vi "FPGAController_v4_check_velocity.vi"() -> ()   [LabVIEW 2015]
uses:
  <vilib>/Utility/miscctls.llb/LVPointTypeDef.ctl
  <vilib>/rvi/interface/nirviOpenFPGA/nirviOpenFPGA.xnode
  <vilib>/rvi/interface/nirviMethod/nirviMethod.xnode
  <vilib>/FPGA/interface/niFpgaViExecutionMode.ctl
  <vilib>/addons/database/NI_Database_API.lvlib
  <vilib>/addons/database/Recordset.llb/Rec Fetch Recordset Data (R).vi
  <vilib>/addons/database/Connection.llb/Conn Execute.vi
  <vilib>/addons/database/Recordset.llb/Rec Destroy - Connection.vi
  <vilib>/addons/database/_DB Variant To Data/Database Variant To Data.xnode
  <vilib>/rvi/interface/nirviReadWriteControl/nirviReadWriteControl.xnode
  NiFpgaLv.dll
  <vilib>/Utility/error.llb/Error Cluster From Error Code.vi
  <vilib>/rvi/errors/niLvFpgaAdjustHostInterfaceError.vi
  <userlib>/_OpenG.lib/file/file.llb/Strip Path Extension - Path__ogtk.vi
  <vilib>/rvi/interface/nirviCloseFPGA/nirviCloseFPGA.xnode
  <vilib>/Utility/file.llb/Write Delimited Spreadsheet (DBL).vi
  <userlib>/_OpenG.lib/comparison/comparison.llb/Boolean Changed__ogtk.vi
  <userlib>/_OpenG.lib/comparison/comparison.llb/DBL Changed__ogtk.vi
  <vilib>/Utility/file.llb/Write Delimited Spreadsheet (string).vi
  FPGA Bitfiles/FPGAnew_FPGATarget_FPGAcodecheckvel_3bbhIfqrdmo.lvbitx
  <vilib>/FPGAPlugInAG/PXIe-7971R/niLvFpga_Close_PXIe-7971R.vi
  <vilib>/FPGAPlugInAG/PXIe-7971R/niLvFpga_Open_PXIe-7971R.vi
panel:
  in  "Tab Control":enum32{"Debugging", "Check Values"}(tab)
  out "Low Mass Limit":fxp<+,31,17>
  out "High Mass Limit":fxp<+,31,17>
  out "Low Charge Limit":i16
  out "High Charge Limit":i16
  out "High velocity count":i32=210
  out "Low velocity count":i32=21000
  out "time":timestamp[](array[timestamp])
  out "Velocity":dbl[](array[numeric])
  out "Filter":i16[](array[numeric])
  out "Time Betwee Shots":dbl
  in  "Min. Time\nBetween Shots (s)":dbl
  in  "Rate Limiting":bool
  out "Update Threshold":bool
  in  "Auto Threshold":bool
  in  "stop":bool
  out "stopping":bool
  in  "One Shot Mode":bool
  out "High Velocity":dbl=100000.0
  out "Low Velocity":dbl=1000.0
  out "Filter 1 Peak":i32=295996
  out "Filter 2 Peak":i32=120664
  out "Filter 3 Peak":i32=46254
  out "Filter 4 Peak":i32=18191
  out "Filter 5 Peak":i32=13910
  out "Filter 6 Peak":i32=9863
  out "Filter 7 Peak":i32=7483
  in  "Zero Peak Values":bool
  in  "Peak-Threshold Factor":dbl=2.0
  in  "Assign Threshold":bool
  in  "Filter1 Threshold":i32=-887988
  in  "Filter2 Threshold":i32=-361992
  in  "Filter3 Threshold":i32=-138762
  in  "Filter4 Threshold":i32=-54306
  in  "Filter5 Threshold":i32=-41730
  in  "Filter6 Threshold":i32=-29358
  in  "Filter7 Threshold":i32=-21165
  out "High Charge Limit (fC)":dbl=100.0
  out "Low Charge Limit (fC)":dbl
  out "Low Mass (kg)":dbl
  out "High Mass (kg)":dbl=inf
  out "Peletron (MV)":dbl=2.0
  in  "Run Mode":bool
  out "error out":errorcluster
  out "Sensitivity":dbl
  out "Last Update:":timestamp
  out "Updating FPGA":bool
  in  "Delay Ring":dbl(ring)=3.15039 items=["Ablation Chamber"=6.45, "LEIL Chamber"=4.318, "Third Detector"=3.15039, "Custom"=0.0]
  in  "Delay Value":dbl=3.0 min=0.0
  in  "Delay Name":string
  in  "Rearm Trigger":bool
  out "Armed":bool
  in  "Add Delay":bool
  in  "Raise Threshold":bool
  in  "Lower Threshold":bool
  out "Del Armed":bool
  # "Settings"
  # "Thresholds"
  # "Peaks"
  # "Independent Variable"
  # "Threshold 1"
  # "Peak 1"
  # "Low Vel."
  # "High Vel."
  # "Threshold 2"
  # "Peak 2"
  # "Low Q (fC)"
  # "High Q (fC)"
  # "Threshold 3"
  # "Peak 3"
  # "Low Mass (kg)"
  # "High Q (fC)"
  # "Threshold 4"
  # "Peak 4"
  # "Sens. (V/pC)"
  # "Peletron (MV)"
  # "Threshold 5"
  # "Peak 5"
  # "Peak Threshold Factor"
  # "Threshold 6"
  # "Peak 6"
  # "Delay Trigger"
  # "Dist. from 2nd Det. (m)"
  # "Name"
  # "Threshold 7"
  # "Peak 7"
  # "Dubugging"
  # "Plate Control While Loop Counter"
  # "Current Value of Running Average"
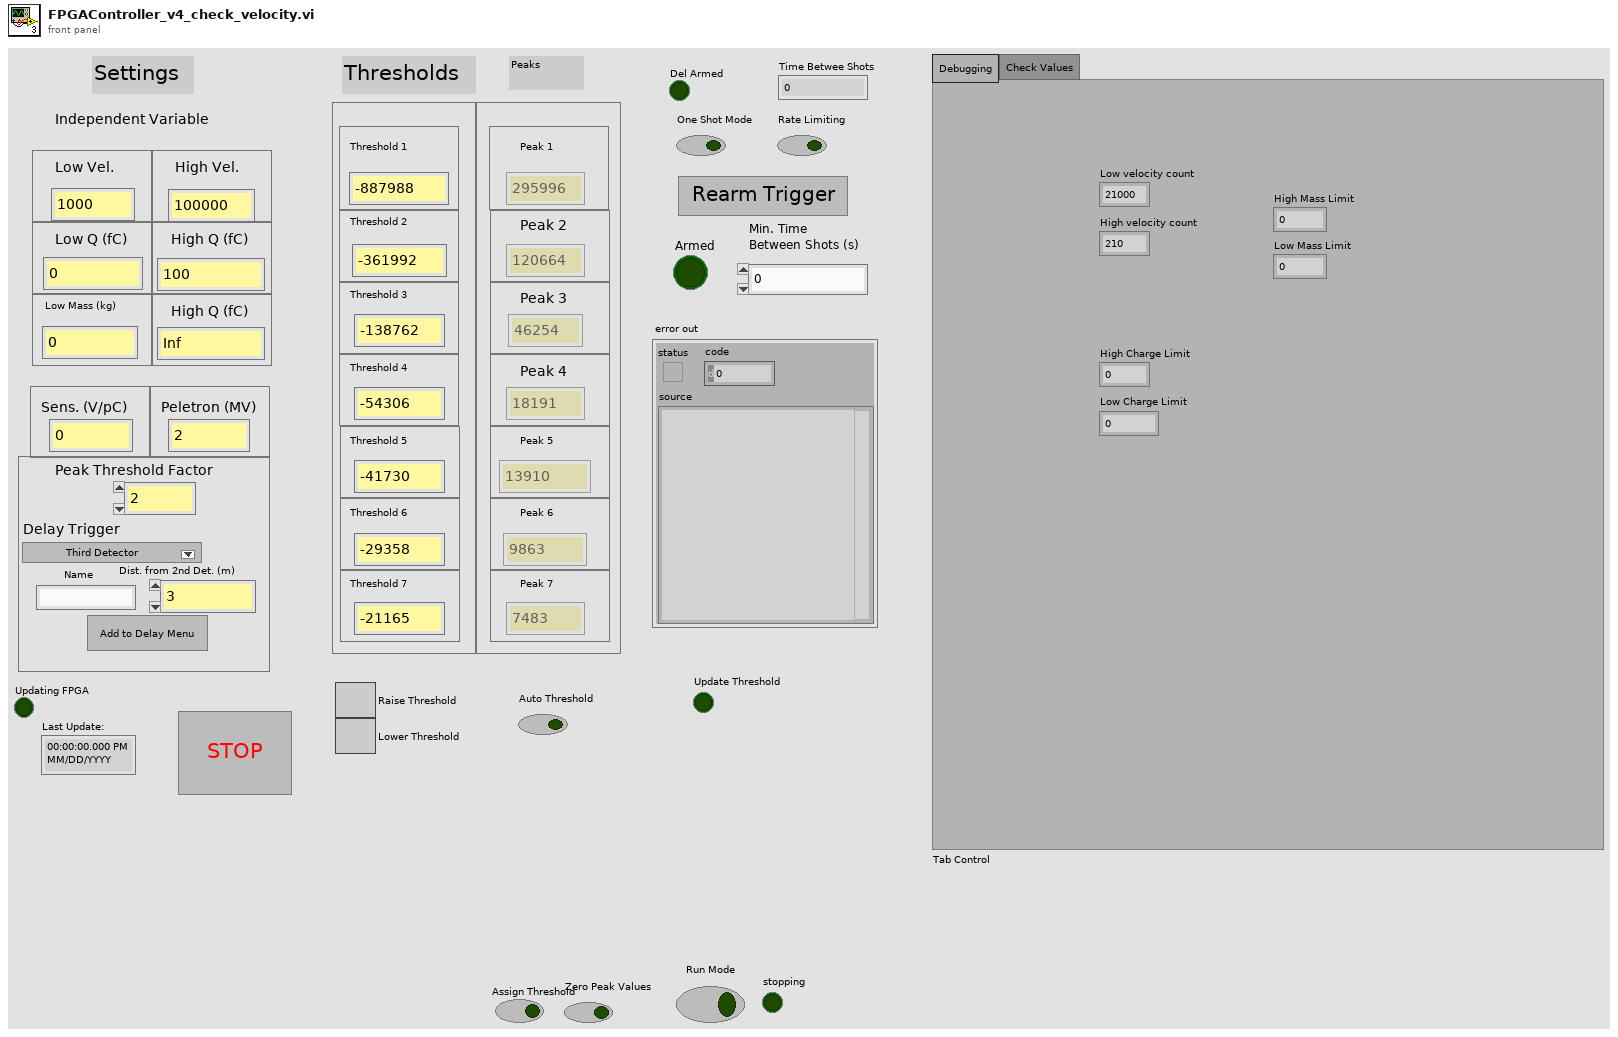
[diagram p1: front panel]
types:
  T1 = typedef "LVPointTypeDef.ctl" = cluster{"Horizontal":i16, "Vertical":i16}
  T2 = enum8{"Enabled", "Disabled", "Disabled and Grayed Out"}
  T3 = typedef "NI_Database_API.lvlib/Conn ObjectReference.ctl" = refnum<k1>
  T4 = cluster{"Filter 1 Peak":i32, "Filter 2 Peak":i32, "Filter 3 Peak":i32, "Filter 4 Peak":i32, "Filter 5 Peak":i32, "Filter 6 Peak":i32, "Filter 7 Peak":i32}
  T5 = typedef "NI_Database_API.lvlib/Rec ObjectReference.ctl" = refnum<k1>
  T6 = typedef "LVStringsAndValuesArrayTypeDef_DBL.ctl" = cluster{"String":string, "Value":dbl}[]
  T7 = cluster{"Numeric":dbl, "Numeric":dbl, "Numeric":dbl, "Numeric":dbl, "Numeric":dbl, "Numeric":dbl, dbl, dbl, "Value":dbl, fxp<+,16,7>, bool}
  T8 = cluster{"Filter 1 Detector 3 Correlation":i32, "Filter 2 Detector 3 Correlation":i32, "Filter 3 Detector 3 Correlation":i32, "Filter 4 Detector 3 Correlation":i32, "Filter 5 Detector 3 Correlation":i32, "Filter 6 Detector 3 Correlation":i32, "Filter 7 Detector 3 Correlation":i32}
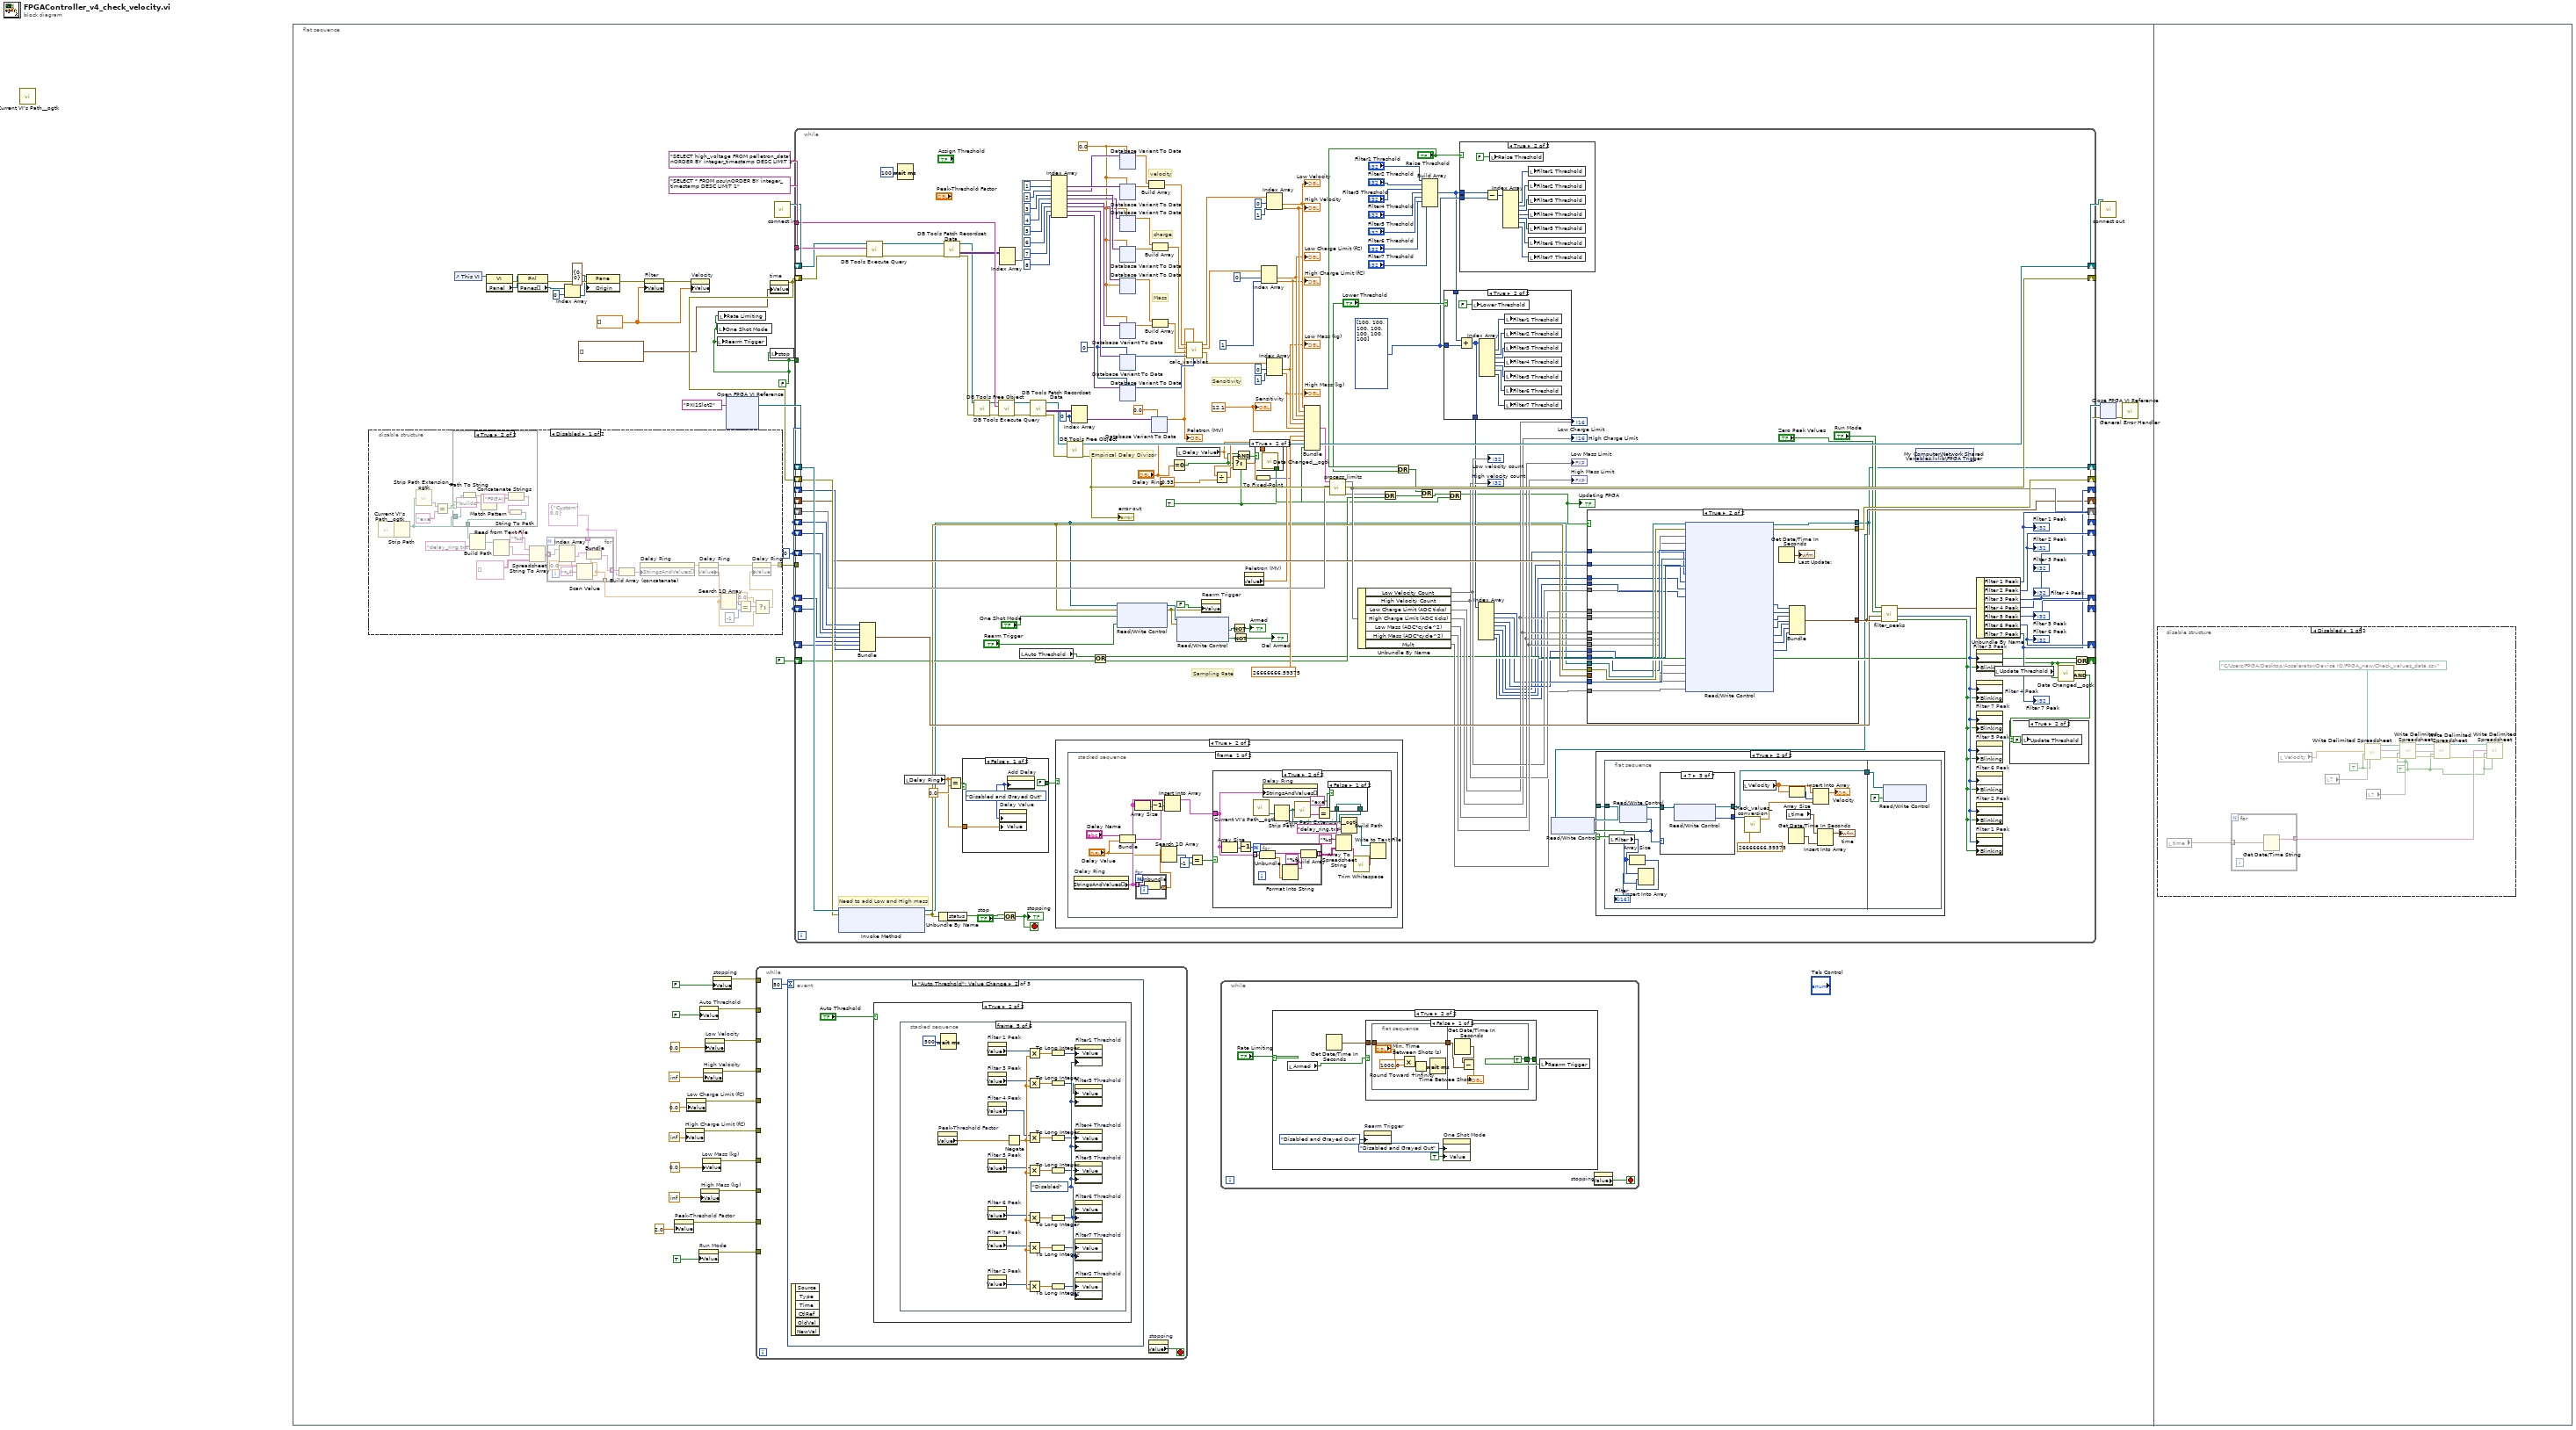
[diagram p0: block diagram]
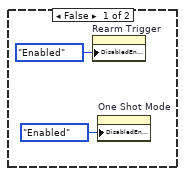
[diagram p4: hidden frame]
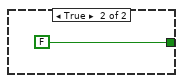
[diagram p5: hidden frame]
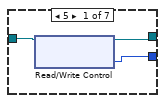
[diagram p7: hidden frame]
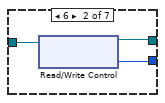
[diagram p8: hidden frame]
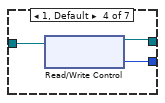
[diagram p9: hidden frame]
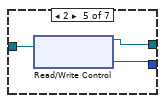
[diagram p10: hidden frame]
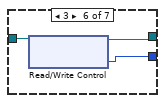
[diagram p11: hidden frame]
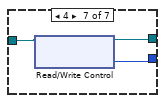
[diagram p12: hidden frame]
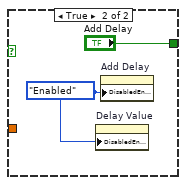
[diagram p17: hidden frame]
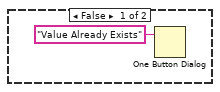
[diagram p19: hidden frame]
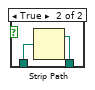
[diagram p20: hidden frame]
diagram:
  n1 = call <userlib>:"Current VI's Path__ogtk.vi"() -> ()  [unwired: 1 in, 1 out]
  n2 = flat-sequence {
    frame #0 {
      w1 = dbl[] [] ("Delay")
      w10 = FALSE
      w45 = 0
      n3 = disable-structure shown="Disabled" {
        disable-tunnel: [w53 _] -> w12
        frame Disabled {
          w62 = cluster{"String":string, "Value":dbl} {"String"="Custom", "Value"=0.0}
          n4 = call <userlib>:"Current VI's Path__ogtk.vi"() -> ("Current VI's Path (+ Relative)"=w71:path)  [unwired: 1 in]
          n5 = Strip Path(path=w71) -> (stripped path=w57:path)  [unwired: 1 out]
          n6 = call-poly <userlib>:"Strip Path Extension__ogtk.vi"("path"=w57) -> ("extension"=w61:string)  [unwired: 1 out]
          n7 = Equal?(x=w61, y="exe") -> (x = y?=w58:bool)
          n8 = case shown="True" w58 {
            tunnel: w57 -> [w80 w87]
            tunnel: [w80 w81] -> w56
            frame False {
            }
            frame True {
              n9 = Path To String(path=w87) -> (string=w86:string)
              n10 = Match Pattern(string=w86, regular expression="builds") -> (before substring=w84:string)  [unwired: 1 in, 3 out]
              n11 = Concatenate Strings(w84, "FPGA\\" ("string")) -> (w82:string)
              n12 = String To Path(string=w82) -> (path=w81:path)
            }
          }
          n13 = Build Path(base path=w56, name or relative path="delay_ring.txt") -> (appended path=w59:path)
          n14 = Read from Text File(file (use dialog)=w59) -> (text=w69:string)  [unwired: 3 in, 3 out]
          n15 = Spreadsheet String To Array(format string="%s", spreadsheet string=w69, array type (2D Dbl)=string[][] []) -> (array=w66:string[][])  [unwired: 1 in]
          n16 = for {
            tunnel: w66 -> [w79] mode=indexing
            tunnel: w62 -> [w77]
            tunnel: [w73] -> w63 mode=indexing
            tunnel: [w72] -> w55 mode=indexing
            n17 = Index Array(array=w79) -> (element #1=w78:string, element #2=w76:string)  [unwired: 2 in]
            n18 = Scan Value(string=w76, format string="%f", default (0 dbl)=0.0) -> (value=w72:dbl)  [unwired: 1 out]
            n19 = Bundle(cluster=w77, "String"=w78, "Value"=w72) -> (w73:cluster{"String":string, "Value":dbl})
          }
          n20 = Build Array (concatenate)(w63, w62) -> (w65:cluster{"String":string, "Value":dbl}[])
          n21 = property on="Delay Ring" class="Ring (strict)"("StringsAndValues[]"=w65) -> (error out=w64:errorcluster)  [unwired: 2 in, 1 out]
          n22 = property on="Delay Ring" class="Ring (strict)"(error in=w64) -> (error out=w54:errorcluster, "Value"=w48:dbl)  [unwired: 1 in, 1 out]
          n23 = Search 1D Array(1D array=w55, element=w48) -> (index of element=w52:i32)  [unwired: 1 in]
          n24 = Equal?(x=w52, y=-1) -> (x = y?=w50:bool)
          n25 = Select(t=0.0, s=w50, f=w48) -> (s? t:f=w49:dbl)
          n26 = property on="Delay Ring" class="Ring (strict)"(error in=w54, "Value"=w49) -> (error out=w53:errorcluster)  [unwired: 1 in, 1 out]
        }
        frame Enabled {
        }
      }
      n27 = control-ref of="This VI"() -> (w22:refnum<vi>)
      n28 = property class="VI"(reference=w22) -> (error out=w21:errorcluster, "Panel"=w20:refnum<vi>)  [unwired: 1 in, 1 out]
      n29 = property class="Pnl"(reference=w20, error in=w21) -> (error out=w19:errorcluster, "Panes[]"=w18:refnum<vi>[])  [unwired: 1 out]
      n30 = Index Array(array=w18, index=0) -> (element=w16:refnum<vi>)
      n31 = property class="Pane"(reference=w16, error in=w19, "Origin"=T1 {"Horizontal"=0, "Vertical"=0}) -> (error out=w3:errorcluster)  [unwired: 1 out]
      n32 = property on="Filter" class="Arr (strict)"(error in=w3, "Value"=w1) -> (error out=w2:errorcluster)  [unwired: 1 in, 1 out]
      n33 = property on="Peak-Threshold Factor" class="DigNum (strict)"("Value"=2.0 ("Peak-Threshold Factor")) -> (error out=w6:errorcluster)  [unwired: 2 in, 1 out]
      n34 = property on="High Charge Limit (fC)" class="DigNum (strict)"("Value"=inf ("High Charge Limit (fC)")) -> (error out=w32:errorcluster)  [unwired: 2 in, 1 out]
      n35 = property on="Low Charge Limit (fC)" class="DigNum (strict)"("Value"=0.0 ("Low Charge Limit (fC)")) -> (error out=w34:errorcluster)  [unwired: 2 in, 1 out]
      n36 = property on="Velocity" class="Arr (strict)"(error in=w2, "Value"=w1) -> ()  [unwired: 1 in, 2 out]
      n37 = property on="Run Mode" class="Bool (strict)"("Value"=TRUE ("Run Mode")) -> (error out=w4:errorcluster)  [unwired: 2 in, 1 out]
      n38 = property on="Auto Threshold" class="Bool (strict)"("Value"=FALSE ("Auto Threshold")) -> (error out=w40:errorcluster)  [unwired: 2 in, 1 out]
      n39 = property on="High Mass (kg)" class="DigNum (strict)"("Value"=inf ("High Mass (kg)")) -> (error out=w28:errorcluster)  [unwired: 2 in, 1 out]
      n40 = property on="Low Mass (kg)" class="DigNum (strict)"("Value"=0.0 ("Low Mass (kg)")) -> (error out=w30:errorcluster)  [unwired: 2 in, 1 out]
      n41 = property on="High Velocity" class="DigNum (strict)"("Value"=inf ("High Velocity")) -> (error out=w36:errorcluster)  [unwired: 2 in, 1 out]
      n42 = property on="Low Velocity" class="DigNum (strict)"("Value"=0.0 ("Low Velocity")) -> (error out=w38:errorcluster)  [unwired: 2 in, 1 out]
      n43 = property on="stopping" class="Bool (strict)"("Value"=FALSE ("stopping")) -> (error out=w42:errorcluster)  [unwired: 2 in, 1 out]
      n44 = local write "Rearm Trigger"(w10) -> ()
      n45 = local write "One Shot Mode"(w10) -> ()
      n46 = local write "Rate Limiting"(w10) -> ()
      n47 = xnode "Open FPGA VI Reference"("resource name"=tag "PXI1Slot2") -> ("FPGA VI Reference Out"=w14:refnum<k20>)  [unwired: 1 in, 1 out]
      n48 = while {
        tunnel: w42 -> [_]
        tunnel: w40 -> [_]
        tunnel: w38 -> [_]
        tunnel: w36 -> [_]
        tunnel: w34 -> [_]
        tunnel: w32 -> [_]
        tunnel: w30 -> [_]
        tunnel: w28 -> [_]
        tunnel: w6 -> [_]
        tunnel: w4 -> [_]
        stop <- w710 stop-if-true
        n49 = event shown="[1] \"Auto Threshold\": Value Change" {
          selector: _ -> [_ _ _]
          dyn-events: _ -> [_ _ _]
          timeout: 50 -> [_ _ _]
          event Timeout {
            n50 = event-data() -> ()  [unwired: 1 in, 2 out]
          }
          event "Auto Threshold": Value Change {
            n51 = event-data() -> ()  [unwired: 1 in, 6 out]
            n52 = case shown="True" "Auto Threshold" {
              frame False {
                w712 = T2."Enabled" ("Disabled")
                n53 = property on="Filter1 Threshold" class="DigNum (strict)"("DisabledEnum"=w712) -> ()  [unwired: 2 in, 2 out]
                n54 = property on="Filter2 Threshold" class="DigNum (strict)"("DisabledEnum"=w712) -> ()  [unwired: 2 in, 2 out]
                n55 = property on="Filter3 Threshold" class="DigNum (strict)"("DisabledEnum"=w712) -> ()  [unwired: 2 in, 2 out]
                n56 = property on="Filter4 Threshold" class="DigNum (strict)"("DisabledEnum"=w712) -> ()  [unwired: 2 in, 2 out]
                n57 = property on="Filter5 Threshold" class="DigNum (strict)"("DisabledEnum"=w712) -> ()  [unwired: 2 in, 2 out]
                n58 = property on="Filter6 Threshold" class="DigNum (strict)"("DisabledEnum"=w712) -> ()  [unwired: 2 in, 2 out]
                n59 = property on="Filter7 Threshold" class="DigNum (strict)"("DisabledEnum"=w712) -> ()  [unwired: 2 in, 2 out]
              }
              frame True {
                n60 = stacked-sequence {
                  frame #0 {
                    n61 = property on="Zero Peak Values" class="Bool (strict)"("Value"=TRUE ("Zero Peak Values")) -> ()  [unwired: 2 in, 2 out]
                    n62 = property on="Run Mode" class="Bool (strict)"("Value"=FALSE ("Run Mode")) -> ()  [unwired: 2 in, 2 out]
                  }
                  frame #1 {
                    n63 = Wait (ms)(milliseconds to wait=u32 2000) -> ()  [unwired: 1 out]
                  }
                  frame #2 {
                    n64 = property on="Zero Peak Values" class="Bool (strict)"("Value"=FALSE ("Zero Peak Values")) -> ()  [unwired: 2 in, 2 out]
                  }
                  frame #3 {
                    n65 = Wait (ms)(milliseconds to wait=u32 8000) -> ()  [unwired: 1 out]
                  }
                  frame #4 {
                    w742 = T2."Disabled" ("Disabled")
                    n66 = property on="Peak-Threshold Factor" class="DigNum (strict)"() -> ("Value"=w727:dbl)  [unwired: 2 in, 2 out]
                    n67 = Wait (ms)(milliseconds to wait=u32 500) -> ()  [unwired: 1 out]
                    n68 = property on="Filter 1 Peak" class="DigNum (strict)"() -> ("Value"=w725:i32)  [unwired: 2 in, 2 out]
                    n69 = property on="Filter 3 Peak" class="DigNum (strict)"() -> ("Value"=w723:i32)  [unwired: 2 in, 2 out]
                    n70 = property on="Filter 4 Peak" class="DigNum (strict)"() -> ("Value"=w722:i32)  [unwired: 2 in, 2 out]
                    n71 = property on="Filter 5 Peak" class="DigNum (strict)"() -> ("Value"=w721:i32)  [unwired: 2 in, 2 out]
                    n72 = property on="Filter 6 Peak" class="DigNum (strict)"() -> ("Value"=w720:i32)  [unwired: 2 in, 2 out]
                    n73 = property on="Filter 7 Peak" class="DigNum (strict)"() -> ("Value"=w719:i32)  [unwired: 2 in, 2 out]
                    n74 = property on="Filter 2 Peak" class="DigNum (strict)"() -> ("Value"=w724:i32)  [unwired: 2 in, 2 out]
                    n75 = Negate(x=w727) -> (-x=w726:dbl)
                    n76 = Multiply(x=w725, y=w726) -> (x*y=w741:dbl)
                    n77 = Multiply(x=w723, y=w726) -> (x*y=w737:dbl)
                    n78 = Multiply(x=w722, y=w726) -> (x*y=w735:dbl)
                    n79 = Multiply(x=w721, y=w726) -> (x*y=w733:dbl)
                    n80 = Multiply(x=w720, y=w726) -> (x*y=w731:dbl)
                    n81 = Multiply(x=w719, y=w726) -> (x*y=w729:dbl)
                    n82 = Multiply(x=w724, y=w726) -> (x*y=w739:dbl)
                    n83 = To Long Integer(number=w741) -> (32bit integer=w740:i32)
                    n84 = To Long Integer(number=w737) -> (32bit integer=w736:i32)
                    n85 = To Long Integer(number=w735) -> (32bit integer=w734:i32)
                    n86 = To Long Integer(number=w733) -> (32bit integer=w732:i32)
                    n87 = To Long Integer(number=w731) -> (32bit integer=w730:i32)
                    n88 = To Long Integer(number=w729) -> (32bit integer=w728:i32)
                    n89 = To Long Integer(number=w739) -> (32bit integer=w738:i32)
                    n90 = property on="Filter1 Threshold" class="DigNum (strict)"("Value"=w740, "DisabledEnum"=w742) -> ()  [unwired: 2 in, 2 out]
                    n91 = property on="Filter3 Threshold" class="DigNum (strict)"("Value"=w736, "DisabledEnum"=w742) -> ()  [unwired: 2 in, 2 out]
                    n92 = property on="Filter4 Threshold" class="DigNum (strict)"("Value"=w734, "DisabledEnum"=w742) -> ()  [unwired: 2 in, 2 out]
                    n93 = property on="Filter5 Threshold" class="DigNum (strict)"("Value"=w732, "DisabledEnum"=w742) -> ()  [unwired: 2 in, 2 out]
                    n94 = property on="Filter6 Threshold" class="DigNum (strict)"("Value"=w730, "DisabledEnum"=w742) -> ()  [unwired: 2 in, 2 out]
                    n95 = property on="Filter7 Threshold" class="DigNum (strict)"("Value"=w728, "DisabledEnum"=w742) -> ()  [unwired: 2 in, 2 out]
                    n96 = property on="Filter2 Threshold" class="DigNum (strict)"("Value"=w738, "DisabledEnum"=w742) -> ()  [unwired: 2 in, 2 out]
                  }
                  frame #5 {
                    n97 = Wait (ms)(milliseconds to wait=u32 500) -> ()  [unwired: 1 out]
                    n98 = property on="Auto Threshold" class="Bool (strict)"("Value"=FALSE ("Auto Threshold")) -> ()  [unwired: 2 in, 2 out]
                    n99 = property on="Run Mode" class="Bool (strict)"("Value"=TRUE ("Run Mode")) -> ()  [unwired: 2 in, 2 out]
                    "Update Threshold" <- TRUE ("Update Threshold")
                  }
                }
              }
            }
          }
          event "Assign Threshold": Value Change {
            n100 = event-data() -> ()  [unwired: 1 in, 6 out]
            n101 = property on="Peak-Threshold Factor" class="DigNum (strict)"() -> ("Value"=w761:dbl)  [unwired: 2 in, 2 out]
            n102 = Wait (ms)(milliseconds to wait=u32 500) -> ()  [unwired: 1 out]
            n103 = property on="Filter 1 Peak" class="DigNum (strict)"() -> ("Value"=w760:i32)  [unwired: 2 in, 2 out]
            n104 = property on="Filter 2 Peak" class="DigNum (strict)"() -> ("Value"=w759:i32)  [unwired: 2 in, 2 out]
            n105 = property on="Filter 3 Peak" class="DigNum (strict)"() -> ("Value"=w758:i32)  [unwired: 2 in, 2 out]
            n106 = property on="Filter 4 Peak" class="DigNum (strict)"() -> ("Value"=w757:i32)  [unwired: 2 in, 2 out]
            n107 = property on="Filter 5 Peak" class="DigNum (strict)"() -> ("Value"=w756:i32)  [unwired: 2 in, 2 out]
            n108 = property on="Filter 6 Peak" class="DigNum (strict)"() -> ("Value"=w755:i32)  [unwired: 2 in, 2 out]
            n109 = property on="Filter 7 Peak" class="DigNum (strict)"() -> ("Value"=w754:i32)  [unwired: 2 in, 2 out]
            n110 = Negate(x=w761) -> (-x=w763:dbl)
            n111 = Multiply(x=w760, y=w763) -> (x*y=w770:dbl)
            n112 = Multiply(x=w759, y=w763) -> (x*y=w768:dbl)
            n113 = Multiply(x=w758, y=w763) -> (x*y=w767:dbl)
            n114 = Multiply(x=w757, y=w763) -> (x*y=w766:dbl)
            n115 = Multiply(x=w756, y=w763) -> (x*y=w765:dbl)
            n116 = Multiply(x=w755, y=w763) -> (x*y=w764:dbl)
            n117 = Multiply(x=w754, y=w763) -> (x*y=w769:dbl)
            n118 = To Long Integer(number=w770) -> (32bit integer=w753:i32)
            n119 = To Long Integer(number=w768) -> (32bit integer=w752:i32)
            n120 = To Long Integer(number=w767) -> (32bit integer=w751:i32)
            n121 = To Long Integer(number=w766) -> (32bit integer=w750:i32)
            n122 = To Long Integer(number=w765) -> (32bit integer=w749:i32)
            n123 = To Long Integer(number=w764) -> (32bit integer=w748:i32)
            n124 = To Long Integer(number=w769) -> (32bit integer=w747:i32)
            n125 = property on="Filter1 Threshold" class="DigNum (strict)"("Value"=w753) -> ()  [unwired: 2 in, 2 out]
            n126 = property on="Filter2 Threshold" class="DigNum (strict)"("Value"=w752) -> ()  [unwired: 2 in, 2 out]
            n127 = property on="Filter3 Threshold" class="DigNum (strict)"("Value"=w751) -> ()  [unwired: 2 in, 2 out]
            n128 = property on="Filter4 Threshold" class="DigNum (strict)"("Value"=w750) -> ()  [unwired: 2 in, 2 out]
            n129 = property on="Filter5 Threshold" class="DigNum (strict)"("Value"=w749) -> ()  [unwired: 2 in, 2 out]
            n130 = property on="Filter6 Threshold" class="DigNum (strict)"("Value"=w748) -> ()  [unwired: 2 in, 2 out]
            n131 = property on="Filter7 Threshold" class="DigNum (strict)"("Value"=w747) -> ()  [unwired: 2 in, 2 out]
          }
        }
        n132 = property on="stopping" class="Bool (strict)"() -> ("Value"=w710:bool)  [unwired: 2 in, 2 out]
      }
      n133 = property on="time" class="Arr (strict)"("Value"=timestamp[] [] ("time")) -> (error out=w9:errorcluster)  [unwired: 2 in, 1 out]
      n134 = local write "stop"(w10) -> ()
      n135 = call "connect in.vi"() -> ("Database Connection"=w23:T3)  [unwired: 7 in, 2 out]
      n136 = while {
        shift-right: [w111] -> w44
        shift-left: w14 -> [w278]
        shift-right: [w274] -> w43
        shift-left: w9 -> [w277]
        shift-right: [w270] -> _
        shift-left: w45 -> [w263]
        shift-right: [w269] -> _
        shift-left: w45 -> [w262]
        shift-right: [w268] -> _
        shift-left: w45 -> [w261]
        shift-right: [w267] -> _
        shift-left: w45 -> [w260]
        shift-right: [w266] -> _
        shift-left: w45 -> [w259]
        shift-right: [w272] -> _
        shift-left: w45 -> [w265]
        shift-right: [w271] -> _
        shift-left: w45 -> [w264]
        tunnel: "SELECT * FROM psu\nORDER BY integer_timestamp DESC LIMIT 1" ("SQL query") -> [w258]
        tunnel: "SELECT high_voltage FROM pelletron_data\nORDER BY integer_timestamp DESC LIMIT 1" ("SQL query") -> [w257]
        shift-right: [w253] -> w24
        shift-left: w23 -> [w256]
        shift-right: [w254] -> _
        shift-left: w9 -> [w255]
        shift-right: [w252] -> _
        shift-left: _ -> [w251]
        shift-right: [w249] -> _
        shift-left: _ -> [w250]
        tunnel: w12 -> [_]
        shift-right: [w154] -> _
        shift-left: FALSE -> [w157]
        tunnel: w10 -> [_]
        stop <- w273 stop-if-true
        w116 = i32[] [100, 100, 100, 100, 100, 100, 100]
        w119 = TRUE
        w205 = 0 ("index (row)")
        w213 = i8 0
        w214 = 0.0
        w179 = 12.1
        # "charge"
        # "Empirical Delay Divisor"
        # "Mass"
        # "velocity"
        # "Sensitivity"
        # "Sampling Rate"
        # "Need to add Low and High mass"
        n137 = xnode "Invoke Method"("FPGA VI Reference In"=w278, "error in"=w277) -> ("FPGA VI Reference Out"=w114:refnum<k20>, "error out"=w173:errorcluster)  [unwired: 1 out]
        n138 = Bundle("Filter 1 Peak"=w265, "Filter 2 Peak"=w264, "Filter 3 Peak"=w263, "Filter 4 Peak"=w262, "Filter 5 Peak"=w261, "Filter 6 Peak"=w260, "Filter 7 Peak"=w259) -> (w245:T4)  [unwired: 1 in]
        n139 = call-poly <vilib>:"DB Tools Execute Query.vi"("error in (no error)"=w255, "SQL query"=w258, "connection reference"=w256) -> ("error out"=w233:errorcluster, "recordset reference"=w234:T5)  [unwired: 5 in]
        n140 = Wait (ms)(milliseconds to wait=u32 100) -> ()  [unwired: 1 out]
        n141 = local read "Delay Ring"() -> (w158:dbl)
        n142 = Unbundle By Name(w173) -> ("status"=w276:bool)
        n143 = call-poly <vilib>:"DB Tools Fetch Recordset Data.vi"("error in (no error)"=w233, "recordset reference"=w234) -> ("error out"=w211:errorcluster, "recordset data"=w224:variant[][], "recordset reference out"=w212:T5)  [unwired: 3 in]
        n144 = Equal?(x=w158, y=0.0) -> (x = y?=w159:bool)
        n145 = case shown="False" w159 {
          tunnel: [FALSE ("Add Delay") "Add Delay"] -> w176
          tunnel: w158 -> [w348 _]
          frame False {
            w349 = T2."Disabled and Grayed Out" ("Disabled")
            n146 = property on="Delay Value" class="DigNum (strict)"("DisabledEnum"=w349, "Value"=w348) -> ()  [unwired: 2 in, 2 out]
            n147 = property on="Add Delay" class="Bool (strict)"("DisabledEnum"=w349) -> ()  [unwired: 2 in, 2 out]
          }
          frame True {
            w350 = T2."Enabled" ("Disabled")
            n148 = property on="Delay Value" class="DigNum (strict)"("DisabledEnum"=w350) -> ()  [unwired: 2 in, 2 out]
            n149 = property on="Add Delay" class="Bool (strict)"("DisabledEnum"=w350) -> ()  [unwired: 2 in, 2 out]
          }
        }
        n150 = call-poly <vilib>:"DB Tools Free Object.vi"("error in (no error)"=w211, "recordset reference"=w212) -> ("error out"=w209:errorcluster, "connection reference"=w210:T3)  [unwired: 8 in]
        n151 = call-poly <vilib>:"DB Tools Execute Query.vi"("error in (no error)"=w209, "SQL query"=w257, "connection reference"=w210) -> ("error out"=w207:errorcluster, "recordset reference"=w208:T5)  [unwired: 5 in]
        n152 = Index Array(array=w224) -> (element=w223:variant[])  [unwired: 2 in]
        n153 = Or(x=w276, y="stop") -> (x .or. y?=w273:bool)
        "stopping" <- w273
        n154 = local read "Auto Threshold"() -> (w155:bool)
        n155 = call-poly <vilib>:"DB Tools Fetch Recordset Data.vi"("error in (no error)"=w207, "recordset reference"=w208) -> ("error out"=w180:errorcluster, "recordset data"=w206:variant[][], "recordset reference out"=w181:T5)  [unwired: 3 in]
        n156 = Index Array(array=w223, index #1=1 ("index"), index #2=2 ("index"), index #3=3 ("index"), index #4=4 ("index"), index #5=5 ("index"), index #6=6 ("index"), index #7=7 ("index"), index #8=8 ("index")) -> (element #1=w222:variant, element #2=w221:variant, element #3=w220:variant, element #4=w219:variant, element #5=w218:variant, element #6=w217:variant, element #7=w216:variant, element #8=w215:variant)
        n157 = case shown="True" w176 {
          frame False {
          }
          frame True {
            n158 = stacked-sequence {
              frame #0 {
                n159 = property on="Delay Ring" class="Ring (strict)"() -> ("StringsAndValues[]"=w354:T6)  [unwired: 2 in, 2 out]
                n160 = Bundle("Delay Name"="Delay Name", "Delay Value"="Delay Value") -> (w359:cluster{"Delay Name":string, "Delay Value":dbl})  [unwired: 1 in]
                n161 = Array Size(array=w354) -> (size(s)=w357:i32)
                n162 = for {
                  tunnel: w354 -> [w364] mode=indexing
                  tunnel: [w363] -> w353 mode=indexing
                  n163 = Unbundle(w364) -> ("Value"=w363:dbl)  [unwired: 1 out]
                }
                n164 = Decrement(x=w357) -> (x-1=w356:i32)
                n165 = Search 1D Array(1D array=w353, element="Delay Value") -> (index of element=w361:i32)  [unwired: 1 in]
                n166 = Insert Into Array(array=w354, index=w356, new element=w359) -> (w358:T6)
                n167 = Equal?(x=w361, y=-1) -> (x = y?=w355:bool)
                n168 = case shown="True" w355 {
                  tunnel: w358 -> [_ w373]
                  frame False {
                    n169 = One Button Dialog(message="Value Already Exists") -> ()  [unwired: 1 in, 1 out]
                  }
                  frame True {
                    n170 = Array Size(array=w373) -> (size(s)=w375:i32)
                    n171 = Decrement(x=w375) -> (x-1=w374:i32)
                    n172 = call <userlib>:"Current VI's Path__ogtk.vi"() -> ("Current VI's Path (+ Relative)"=w379:path)  [unwired: 1 in]
                    n173 = for {
                      N: w374 -> [_]
                      tunnel: w373 -> [w389] mode=indexing
                      tunnel: [w384] -> w376 mode=indexing
                      n174 = Unbundle(w389) -> ("String"=w385:string, "Value"=w388:dbl)
                      n175 = Format Into String(format string="%f", w388) -> (resulting string=w386:string)  [unwired: 2 in, 1 out]
                      n176 = Build Array(w385, w386) -> (w384:string[])
                    }
                    n177 = property on="Delay Ring" class="Ring (strict)"("StringsAndValues[]"=w373) -> ()  [unwired: 2 in, 2 out]
                    n178 = Strip Path(path=w379) -> (stripped path=w367:path)  [unwired: 1 out]
                    n179 = call-poly <userlib>:"Strip Path Extension__ogtk.vi"("path"=w367) -> ("extension"=w370:string)  [unwired: 1 out]
                    n180 = Equal?(x="exe", y=w370) -> (x = y?=w368:bool)
                    n181 = case shown="False" w368 {
                      tunnel: w367 -> [w381 w383]
                      tunnel: [w381 w382] -> w366
                      frame False {
                      }
                      frame True {
                        n182 = Strip Path(path=w383) -> (stripped path=w382:path)  [unwired: 1 out]
                      }
                    }
                    n183 = Array To Spreadsheet String(array=w376, 3:"%s" ("format string")) -> (spreadsheet string=w372:string)  [unwired: 1 in]
                    n184 = Build Path(base path=w366, name or relative path="delay_ring.txt") -> (appended path=w377:path)
                    n185 = call <vilib>:"Trim Whitespace.vi"("string"=w372) -> ("trimmed string"=w371:string)  [unwired: 1 in]
                    n186 = Write to Text File(file (use dialog)=w377, text=w371) -> ()  [unwired: 2 in, 3 out]
                  }
                }
              }
              frame #1 {
                n187 = property on="Add Delay" class="Bool (strict)"("Value"=FALSE ("Add Delay")) -> ()  [unwired: 2 in, 2 out]
              }
            }
          }
        }
        n188 = call-poly <vilib>:"DB Tools Free Object.vi"("error in (no error)"=w180, "recordset reference"=w181) -> ("error out"=w254:errorcluster, "connection reference"=w253:T3)  [unwired: 8 in]
        "error out" <- w254
        n189 = Index Array(array=w206, index (row)=w205, index (col)=w205) -> (element=w204:variant)
        n190 = Or(x=w155, y=w157) -> (x .or. y?=w156:bool)
        n191 = xnode "Read/Write Control"("FPGA VI Reference In"=w114, "error in"=w173, "One Shot"="One Shot Mode", "Reset One Shot"="Rearm Trigger") -> ("FPGA VI Reference Out"=w167:refnum<k20>, "error out"=w166:errorcluster)
        n192 = xnode "Database Variant To Data"("database variant"=w221, "type"=w214) -> ("data"=w130:dbl)  [unwired: 1 in, 1 out]
        n193 = xnode "Database Variant To Data"("database variant"=w222, "type"=w214) -> ("data"=w131:dbl)  [unwired: 1 in, 1 out]
        n194 = xnode "Database Variant To Data"("database variant"=w219, "type"=w214) -> ("data"=w129:dbl)  [unwired: 1 in, 1 out]
        n195 = xnode "Database Variant To Data"("database variant"=w220, "type"=w214) -> ("data"=w128:dbl)  [unwired: 1 in, 1 out]
        n196 = xnode "Database Variant To Data"("database variant"=w217, "type"=w214) -> ("data"=w127:dbl)  [unwired: 1 in, 1 out]
        n197 = xnode "Database Variant To Data"("database variant"=w218, "type"=w214) -> ("data"=w126:dbl)  [unwired: 1 in, 1 out]
        n198 = xnode "Database Variant To Data"("database variant"=w216, "type"=w213) -> ("data"=w198:i8)  [unwired: 1 in, 1 out]
        n199 = xnode "Database Variant To Data"("database variant"=w215, "type"=w213) -> ("data"=w197:i8)  [unwired: 1 in, 1 out]
        n200 = Build Array(w130, w131) -> (w201:dbl[])
        n201 = xnode "Database Variant To Data"("database variant"=w204, "type"=0.0) -> ("data"=w125:dbl)  [unwired: 1 in, 1 out]
        "Peletron (MV)" <- w125
        n202 = Build Array(w129, w128) -> (w200:dbl[])
        n203 = Build Array(w127, w126) -> (w199:dbl[])
        n204 = Equal To 0?(x="Delay Ring") -> (x = 0?=w124:bool)
        n205 = xnode "Read/Write Control"("FPGA VI Reference In"=w167, "error in"=w166) -> ("Not Armed?"=w165:bool, "Del Not Armed?"=w118:bool)  [unwired: 2 out]
        n206 = local read "Delay Value"() -> (w123:dbl)
        n207 = call "calc_variables.vi"("var2"=w197, "Peletron"=w125, "var1"=w198, "Mass"=w199, "Charge"=w200, "Velocity"=w201) -> ("Mass out"=w190:dbl[], "Charge out"=w193:dbl[], "Velocity out"=w196:dbl[])  [unwired: 3 in]
        n208 = property on="Rearm Trigger" class="Bool (strict)"(error in=w166, "Value"=FALSE ("Rearm Trigger")) -> ()  [unwired: 1 in, 2 out]
        n209 = Divide(x="Delay Ring", y=0.93) -> (x/y=w163:dbl)
        n210 = Select(t=w123, s=w124, f=w163) -> (s? t:f=w162:dbl)
        n211 = Not(x=w165) -> (.not. x?=→"Armed":bool)
        n212 = Not(x=w118) -> (.not. x?=→"Del Armed":bool)
        n213 = And(x=w124, y=w119) -> (x .and. y?=w120:bool)
        n214 = property on="Peletron (MV)" class="DigNum (strict)"() -> ("Value"=w202:dbl)  [unwired: 2 in, 2 out]
        n215 = case shown="True" w120 {
          selector: w120 -> [w320 _]
          tunnel: w123 -> [_ w322]
          tunnel: [w320 w321] -> w121
          frame False {
          }
          frame True {
            n216 = call-poly <userlib>:"Data Changed__ogtk.vi"("DBL"=w322) -> ("Changed"=w321:bool)
          }
        }
        n217 = To Fixed-Point(number=w162) -> (fixed-point=w175:fxp<+,16,7>)  [unwired: 1 in]
        n218 = Index Array(array=w193, index #1=0 ("index"), index #2=1 ("index")) -> (element #1=w185:dbl, element #2=w184:dbl)
        "High Charge Limit (fC)" <- w184
        "Low Charge Limit (fC)" <- w185
        n219 = Index Array(array=w196, index #1=0 ("index"), index #2=1 ("index")) -> (element #1=w187:dbl, element #2=w186:dbl)
        "High Velocity" <- w186
        "Low Velocity" <- w187
        n220 = Index Array(array=w190, index #1=0 ("index"), index #2=1 ("index")) -> (element #1=w183:dbl, element #2=w182:dbl)
        "Low Mass (kg)" <- w183
        "High Mass (kg)" <- w182
        n221 = Bundle("Numeric"=w187, "Numeric"=w186, "Numeric"=w185, "Numeric"=w184, "Numeric"=w183, "Numeric"=w182, w179, 26666666.59375, "Value"=w202, w175, w119) -> (w244:T7)  [unwired: 1 in]
        n222 = call "process_limits.vi"(10:w251, 11:w244) -> (0:w178, 3:w252)  [unwired: 8 in]
        n223 = Unbundle By Name(w252) -> ("Low Velocity Count"=w240, "High Velocity Count"=w239, "Low Charge Limit (ADC ticks)"=w237, "High Charge Limit (ADC ticks)"=w238, "Low Mass (ADC*cycle^2)"=w242, "High Mass (ADC*cycle^2)"=w243, "Mult"=w174)
        "Low velocity count" <- w240
        "High velocity count" <- w239
        "High Charge Limit" <- w238
        "Low Charge Limit" <- w237
        "High Mass Limit" <- w243
        "Low Mass Limit" <- w242
        n224 = Or(x=w178, y=w156) -> (x .or. y?=w161:bool)
        n225 = Or(x="Raise Threshold", y="Lower Threshold") -> (x .or. y?=w132:bool)
        n226 = Or(x=w132, y=w161) -> (x .or. y?=w133:bool)
        n227 = Build Array("Filter1 Threshold", "Filter2 Threshold", "Filter3 Threshold", "Filter4 Threshold", "Filter5 Threshold", "Filter6 Threshold", "Filter7 Threshold") -> (w115:i32[])
        n228 = case shown="True" "Lower Threshold" {
          tunnel: w115 -> [w323 w334]
          tunnel: w116 -> [_ w333]
          tunnel: [w323 w324] -> w146
          frame False {
          }
          frame True {
            n229 = Add(x=w334, y=w333) -> (x+y=w324:i32[])
            n230 = local write "Lower Threshold"(FALSE ("Lower Threshold")) -> ()
            n231 = Index Array(array=w324) -> (element #1=w331:i32, element #2=w330:i32, element #3=w329:i32, element #4=w328:i32, element #5=w327:i32, element #6=w326:i32, element #7=w325:i32)  [unwired: 7 in]
            n232 = local write "Filter1 Threshold"(w331) -> ()
            n233 = local write "Filter2 Threshold"(w330) -> ()
            n234 = local write "Filter3 Threshold"(w329) -> ()
            n235 = local write "Filter4 Threshold"(w328) -> ()
            n236 = local write "Filter5 Threshold"(w327) -> ()
            n237 = local write "Filter6 Threshold"(w326) -> ()
            n238 = local write "Filter7 Threshold"(w325) -> ()
          }
        }
        n239 = Or(x=w133, y=w121) -> (x .or. y?=w122:bool)
        "Updating FPGA" <- w122
        n240 = case shown="True" "Raise Threshold" {
          tunnel: w115 -> [_ w345]
          tunnel: w116 -> [_ w335]
          frame False {
          }
          frame True {
            n241 = Subtract(x=w345, y=w335) -> (x-y=w336:i32[])
            n242 = local write "Raise Threshold"(FALSE ("Raise Threshold")) -> ()
            n243 = Index Array(array=w336) -> (element #1=w343:i32, element #2=w342:i32, element #3=w341:i32, element #4=w340:i32, element #5=w339:i32, element #6=w338:i32, element #7=w337:i32)  [unwired: 7 in]
            n244 = local write "Filter1 Threshold"(w343) -> ()
            n245 = local write "Filter2 Threshold"(w342) -> ()
            n246 = local write "Filter3 Threshold"(w341) -> ()
            n247 = local write "Filter4 Threshold"(w340) -> ()
            n248 = local write "Filter5 Threshold"(w339) -> ()
            n249 = local write "Filter6 Threshold"(w338) -> ()
            n250 = local write "Filter7 Threshold"(w337) -> ()
          }
        }
        n251 = Index Array(array=w146) -> (element #1=w149:i32, element #2=w147:i32, element #3=w144:i32, element #4=w142:i32, element #5=w140:i32, element #6=w138:i32, element #7=w136:i32)  [unwired: 7 in]
        n252 = case shown="True" w122 {
          tunnel: w114 -> [w392 w420]
          tunnel: w173 -> [w393 w419]
          tunnel: [w392 w418] -> w111
          tunnel: [w393 w417] -> w274
          tunnel: w149 -> [_ w416]
          tunnel: w147 -> [_ w415]
          tunnel: w144 -> [_ w414]
          tunnel: w142 -> [_ w413]
          tunnel: w140 -> [_ w412]
          tunnel: w138 -> [_ w411]
          tunnel: w136 -> [_ w410]
          tunnel: [w391 w396] -> w249
          tunnel: w243 -> [_ w402]
          tunnel: w242 -> [_ w401]
          tunnel: w240 -> [_ w400]
          tunnel: w239 -> [_ w399]
          tunnel: w238 -> [_ w398]
          tunnel: w237 -> [_ w397]
          tunnel: w250 -> [w391 _]
          tunnel: w174 -> [_ w394]
          frame False {
          }
          frame True {
            n253 = xnode "Read/Write Control"("FPGA VI Reference In"=w420, "error in"=w419, "Low Velocity Count"=w400, "High Velocity Count"=w399, "Filter 1 threshold"=w416, "Filter 2 threshold"=w415, "Filter 3 threshold"=w414, "Filter 4 threshold"=w413, "Filter 5 threshold"=w412, "Filter 6 threshold"=w411, "Filter 7 threshold"=w410, "High Charge Limit"=w398, "Low Charge Limit"=w397, "High Mass Limit"=w402, "Low Mass Limit"=w401, "Mult1"=w394) -> ("FPGA VI Reference Out"=w418:refnum<k20>, "error out"=w417:errorcluster, "Filter 1 Detector 3 Correlation"=w409:i32, "Filter 2 Detector 3 Correlation"=w408:i32, "Filter 3 Detector 3 Correlation"=w407:i32, "Filter 4 Detector 3 Correlation"=w406:i32, "Filter 5 Detector 3 Correlation"=w405:i32, "Filter 6 Detector 3 Correlation"=w404:i32, "Filter 7 Detector 3 Correlation"=w403:i32)
            n254 = Get Date/Time In Seconds() -> (seconds since 1Jan1904=→"Last Update:":timestamp)
            n255 = Bundle("Filter 1 Detector 3 Correlation"=w409, "Filter 2 Detector 3 Correlation"=w408, "Filter 3 Detector 3 Correlation"=w407, "Filter 4 Detector 3 Correlation"=w406, "Filter 5 Detector 3 Correlation"=w405, "Filter 6 Detector 3 Correlation"=w404, "Filter 7 Detector 3 Correlation"=w403) -> (w396:T8)  [unwired: 1 in]
          }
        }
        n256 = xnode "Read/Write Control"("FPGA VI Reference In"=w111) -> ("FPGA VI Reference Out"=w112:refnum<k20>, "Check Data?"=w113:bool)  [unwired: 1 in, 1 out]
        n257 = case shown="True" w113 {
          tunnel: w112 -> [_ w280]
          frame False {
          }
          frame True {
            n258 = flat-sequence {
              tunnel: w280 -> [w296]
              tunnel: [w281] -> w279
              tunnel: w279 -> [w319]
              frame #0 {
                n259 = local read "Filter"() -> (w282:i16[])
                n260 = xnode "Read/Write Control"("FPGA VI Reference In"=w296) -> ("FPGA VI Reference Out"=w295:refnum<k20>, "Filter"=w284:i16)  [unwired: 1 in, 1 out]
                n261 = Array Size(array=w282) -> (size(s)=w285:i32)
                n262 = Insert Into Array(array=w282, index=w285, new element=w284) -> (→"Filter":i16[])
                n263 = case shown="7" w284 {
                  tunnel: w295 -> [w299 w302 w305 w308 w311 w314 w317]
                  tunnel: [w298 w301 w304 w307 w310 w313 w316] -> w290
                  tunnel: [w297 w300 w303 w306 w309 w312 w315] -> w281
                  frame 5 {
                    n264 = xnode "Read/Write Control"("FPGA VI Reference In"=w299) -> ("FPGA VI Reference Out"=w297:refnum<k20>, "Vel Count 5"=w298:i32)  [unwired: 1 in, 1 out]
                  }
                  frame 6 {
                    n265 = xnode "Read/Write Control"("FPGA VI Reference In"=w302) -> ("FPGA VI Reference Out"=w300:refnum<k20>, "Vel Count 6"=w301:i32)  [unwired: 1 in, 1 out]
                  }
                  frame 7 {
                    n266 = xnode "Read/Write Control"("FPGA VI Reference In"=w305) -> ("FPGA VI Reference Out"=w303:refnum<k20>, "Vel Count 7"=w304:i32)  [unwired: 1 in, 1 out]
                  }
                  frame 1, Default {
                    n267 = xnode "Read/Write Control"("FPGA VI Reference In"=w308) -> ("FPGA VI Reference Out"=w306:refnum<k20>, "Vel Count 1"=w307:i32)  [unwired: 1 in, 1 out]
                  }
                  frame 2 {
                    n268 = xnode "Read/Write Control"("FPGA VI Reference In"=w311) -> ("FPGA VI Reference Out"=w309:refnum<k20>, "Vel Count 2"=w310:i32)  [unwired: 1 in, 1 out]
                  }
                  frame 3 {
                    n269 = xnode "Read/Write Control"("FPGA VI Reference In"=w314) -> ("FPGA VI Reference Out"=w312:refnum<k20>, "Vel Count 3"=w313:i32)  [unwired: 1 in, 1 out]
                  }
                  frame 4 {
                    n270 = xnode "Read/Write Control"("FPGA VI Reference In"=w317) -> ("FPGA VI Reference Out"=w315:refnum<k20>, "Vel Count 4"=w316:i32)  [unwired: 1 in, 1 out]
                  }
                }
                n271 = local read "Velocity"() -> (w286:dbl[])
                n272 = call "Check_values_conversion.vi"("Sampling Rate"=26666666.59375, "Velocity  Count"=w290) -> ("Measured Velocity"=w288:dbl)  [unwired: 2 in, 2 out]
                n273 = local read "time"() -> (w291:timestamp[])
                n274 = Get Date/Time In Seconds() -> (seconds since 1Jan1904=w293:timestamp)
                n275 = Array Size(array=w286) -> (size(s)=w287:i32)
                n276 = Insert Into Array(array=w286, index=w287, new element=w288) -> (→"Velocity":dbl[])
                n277 = Insert Into Array(array=w291, new element=w293) -> (→"time":timestamp[])  [unwired: 1 in]
              }
              frame #1 {
                n278 = xnode "Read/Write Control"("FPGA VI Reference In"=w319, "Check Data?"=FALSE) -> ()  [unwired: 1 in, 2 out]
              }
            }
          }
        }
        n279 = call "filter_peaks.vi"("Correlation cluster"=w249, "Filter peak cluster"=w245, "Zero out"="Zero Peak Values", "Run Mode"="Run Mode") -> ("Blinking"=w236:bool, "status"=w241:T2, "Filter peak output"=w246:T4)  [unwired: 5 in]
        n280 = shared-variable "My Computer\\Network Shared Variables.lvlib\\FPGA Trigger"() -> ()  [unwired: 1 in, 2 out]
        n281 = Unbundle By Name(w246) -> ("Filter 1 Peak"=w272:i32, "Filter 2 Peak"=w271:i32, "Filter 3 Peak"=w270:i32, "Filter 4 Peak"=w269:i32, "Filter 5 Peak"=w268:i32, "Filter 6 Peak"=w267:i32, "Filter 7 Peak"=w266:i32)
        "Filter 1 Peak" <- w272
        "Filter 2 Peak" <- w271
        "Filter 3 Peak" <- w270
        "Filter 4 Peak" <- w269
        "Filter 5 Peak" <- w268
        "Filter 6 Peak" <- w267
        "Filter 7 Peak" <- w266
        n282 = property on="Filter 3 Peak" class="DigNum (strict)"("DisabledEnum"=w241, "Blinking"=w236) -> ()  [unwired: 2 in, 2 out]
        n283 = property on="Filter 4 Peak" class="DigNum (strict)"("DisabledEnum"=w241, "Blinking"=w236) -> ()  [unwired: 2 in, 2 out]
        n284 = property on="Filter 7 Peak" class="DigNum (strict)"("DisabledEnum"=w241, "Blinking"=w236) -> ()  [unwired: 2 in, 2 out]
        n285 = property on="Filter 5 Peak" class="DigNum (strict)"("DisabledEnum"=w241, "Blinking"=w236) -> ()  [unwired: 2 in, 2 out]
        n286 = property on="Filter 6 Peak" class="DigNum (strict)"("DisabledEnum"=w241, "Blinking"=w236) -> ()  [unwired: 2 in, 2 out]
        n287 = property on="Filter 2 Peak" class="DigNum (strict)"("DisabledEnum"=w241, "Blinking"=w236) -> ()  [unwired: 2 in, 2 out]
        n288 = property on="Filter 1 Peak" class="DigNum (strict)"("DisabledEnum"=w241, "Blinking"=w236) -> ()  [unwired: 2 in, 2 out]
        n289 = local read "Update Threshold"() -> (w152:bool)
        n290 = call-poly <userlib>:"Data Changed__ogtk.vi"("Boolean"=w152) -> ("Changed"=w153:bool)
        n291 = And(x=w153, y=w152) -> (x .and. y?=w151:bool)
        n292 = case shown="True" w151 {
          frame False {
          }
          frame True {
            n293 = local write "Update Threshold"(FALSE ("Update Threshold")) -> ()
          }
        }
        n294 = Or(x=w155, y=w152) -> (x .or. y?=w154:bool)
        "Sensitivity" <- w179
      }
      n295 = while {
        stop <- w89 stop-if-true
        n296 = case shown="True" "Rate Limiting" {
          frame False {
            n297 = property on="Rearm Trigger" class="Bool (strict)"("DisabledEnum"=T2."Enabled" ("Disabled")) -> ()  [unwired: 2 in, 2 out]
            n298 = property on="One Shot Mode" class="Bool (strict)"("DisabledEnum"=T2."Enabled" ("Disabled")) -> ()  [unwired: 2 in, 2 out]
          }
          frame True {
            n299 = local read "Armed"() -> (w93:bool)
            n300 = Get Date/Time In Seconds() -> (seconds since 1Jan1904=w92:timestamp)
            n301 = property on="Rearm Trigger" class="Bool (strict)"("DisabledEnum"=T2."Disabled and Grayed Out" ("Disabled")) -> ()  [unwired: 2 in, 2 out]
            n302 = case shown="False" w93 {
              tunnel: [w100 FALSE] -> w97
              tunnel: w92 -> [w99 _]
              frame False {
                n303 = flat-sequence {
                  tunnel: w99 -> [w101]
                  tunnel: [w101] -> w98
                  tunnel: [TRUE] -> w100
                  tunnel: w98 -> [w107]
                  frame #0 {
                    n304 = Multiply(x="Min. Time\nBetween Shots (s)", y=1000.0) -> (x*y=w104:dbl)
                    n305 = Round Toward +Infinity(x=w104) -> (ceil(x): smallest int >= x=w102:dbl)
                    n306 = Wait (ms)(milliseconds to wait=w102) -> ()  [unwired: 1 out]
                  }
                  frame #1 {
                    n307 = Get Date/Time In Seconds() -> (seconds since 1Jan1904=w108:timestamp)
                    n308 = Subtract(x=w108, y=w107) -> (x-y=→"Time Betwee Shots":dbl)
                  }
                }
              }
              frame True {
              }
            }
            n309 = property on="One Shot Mode" class="Bool (strict)"("DisabledEnum"=T2."Disabled and Grayed Out" ("Disabled"), "Value"=TRUE ("One Shot Mode")) -> ()  [unwired: 2 in, 2 out]
            n310 = local write "Rearm Trigger"(w97) -> ()
          }
        }
        n311 = property on="stopping" class="Bool (strict)"() -> ("Value"=w89:bool)  [unwired: 2 in, 2 out]
      }
      n312 = call "connect out.vi"("connection reference"=w24) -> ()  [unwired: 10 in, 1 out]
      n313 = xnode "Close FPGA VI Reference"("FPGA VI Reference In"=w44, "error in"=w43) -> ("error out"=w46:errorcluster)
      n314 = call <vilib>:"General Error Handler.vi"("error in (no error)"=w46) -> ()  [unwired: 10 in, 5 out]
    }
    frame #1 {
      n315 = disable-structure shown="Disabled" {
        frame Disabled {
          w772 = TRUE ("transpose? (F)")
          w771 = TRUE ("append to file? (F)")
          n316 = local read "time"() -> (w784:timestamp[])
          n317 = for {
            tunnel: w784 -> [w786] mode=indexing
            tunnel: [w785] -> w783 mode=indexing
            n318 = Get Date/Time String(seconds (now)=w786) -> (date string=w785:string)  [unwired: 2 in, 1 out]
          }
          n319 = local read "Velocity"() -> (w775:dbl[])
          n320 = local read item#-1() -> (w774)
          n321 = call-poly <vilib>:"Write Delimited Spreadsheet.vi"("file path (dialog if empty)"=path "C:/Users/FPGA/Desktop/Accelerator/Device IO/FPGA_new/Check_values_data.csv", "1D data"=w775, "append to file? (F)"=w771, "transpose? (F)"=w771) -> ("new file path (Not A Path if cancelled)"=w781:path, "error out"=w778:errorcluster)  [unwired: 10 in]
          n322 = local read item#-1() -> (w773)
          n323 = call-poly <vilib>:"Write Delimited Spreadsheet.vi"("file path (dialog if empty)"=w781, "1D data"=w774, "append to file? (F)"=w772, "error in (no error)"=w778, "transpose? (F)"=w772) -> ("new file path (Not A Path if cancelled)"=w780:path, "error out"=w777:errorcluster)  [unwired: 9 in]
          n324 = call-poly <vilib>:"Write Delimited Spreadsheet.vi"("file path (dialog if empty)"=w780, "1D data"=w773, "append to file? (F)"=w772, "error in (no error)"=w777) -> ("new file path (Not A Path if cancelled)"=w779:path, "error out"=w776:errorcluster)  [unwired: 10 in]
          n325 = call-poly <vilib>:"Write Delimited Spreadsheet.vi"("file path (dialog if empty)"=w779, "1D data"=w783, "append to file? (F)"=w772, "error in (no error)"=w776, "transpose? (F)"=w772) -> ()  [unwired: 9 in, 2 out]
        }
        frame Enabled {
        }
      }
    }
  }
